vi "Set_To_Idle_State.vi"(6 "Standalone?":bool, 8 "Error In":errorcluster, 9 "GEA2 Reference In":refnum<k24>, 10 "GEA Inputs":T1 {"Destination" format="%.0x"; "Source" format="%.0x"}, 11 "Device Selected":i32) -> (0 "Error Out":errorcluster, 1 "GEA2 Reference Out":refnum<k24>, 3 "Press Power Key":bool)   [LabVIEW 2014]
uses:
  Common/LabVIEW GEA2 Toolkit/LabVIEW_GEA2_Toolkit.lvlibp/type defs/Source_Destination.ctl
  Common/LabVIEW GEA2 Toolkit/LabVIEW_GEA2_Toolkit.lvlibp/type defs/ERD Read Data In.ctl
  Common/LabVIEW GEA2 Toolkit/LabVIEW_GEA2_Toolkit.lvlibp/type defs/Data Type.ctl
  type defs/HEUI Switches.ctl
  Common/LabVIEW GEA2 Toolkit/LabVIEW_GEA2_Toolkit.lvlibp
  C:/Automation/DLLs/PC Tools .NET/GeaCommunication.dll
panel:
  out "Status 2000":string
  # "2015 Dryer: Set to Idle State"
  # "Send Status ERD 2000.\nIf not in Idle (0), press Power key.\nIf in Idle, do nothing."
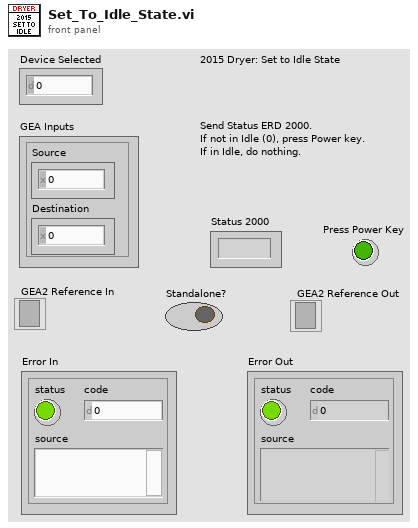
[diagram p1: front panel]
types:
  T1 = typedef "LabVIEW_GEA2_Toolkit.lvlibp/Source_Destination.ctl" = cluster{"Source":u8, "Destination":u8}
  T2 = typedef "LabVIEW_GEA2_Toolkit.lvlibp/ERD Read Data In.ctl" = cluster{"ERD Number":u16, "Data Type":T3}
  T3 = typedef "LabVIEW_GEA2_Toolkit.lvlibp/Data Type.ctl" = enum16{"string", "boolean", "uint8_t", "uint16_t", "uint32_t", "uint64_t", "int8_t", "int16_t", "int32_t", "int64_t"}
  T4 = typedef "LabVIEW_GEA2_Toolkit.lvlibp/ERD Read Data Out.ctl" = cluster{"ERD Number":u16, "Data":string}
  T5 = typedef "HEUI Switches.ctl" = enum16{"Switch Off /  Reset", "SW201 - My Cycle", "SW202 - Delay Dry", "SW203 - Signal / Volume", "SW204 - Damp Alert", "SW205 - Temp", "SW206 - Ext Tumble", "SW207 - Dryness Level", "SW208 -  (-) Time", "SW209 - Time", "SW210 - (+) Time", "SW211 - eDry ", "SW212 - null", "SW213 - Power", "SW214 - Start / Pause"}
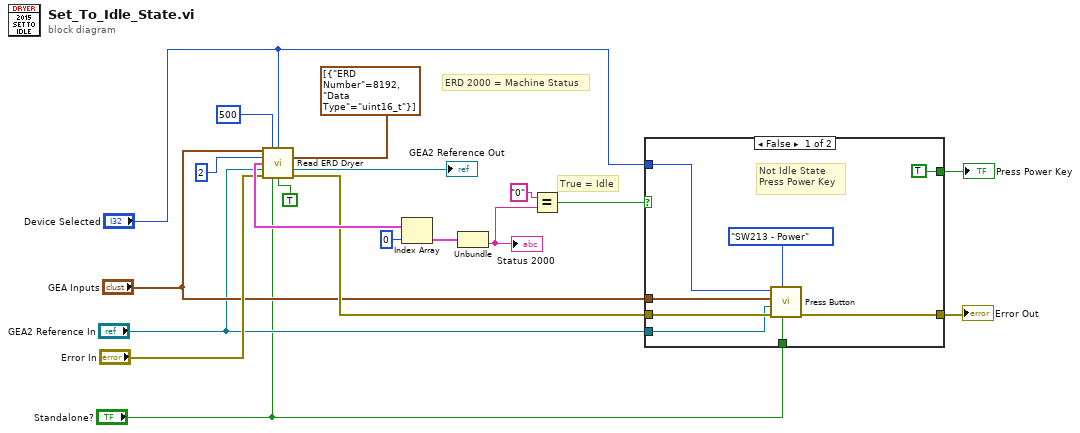
[diagram p0: block diagram]
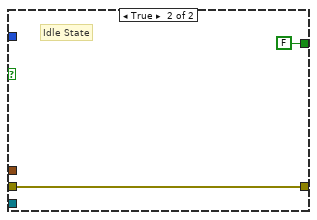
[diagram p2: hidden frame]
diagram:
  # "ERD 2000 = Machine Status"
  # "True = Idle"
  n1 = call "Read ERD Dryer.vi"("GEA Inputs"="GEA Inputs", "Read Timeout (ms)"=u32 500, "Device Selected"="Device Selected", "Retry Count"=2, "Read ERD List"=T2[] [{"ERD Number"=8192, "Data Type"=enum."uint16_t"}], "GEA2 Reference In"="GEA2 Reference In", "Error In"="Error In", "Standalone?"="Standalone?", "Verify ERD Response?"=TRUE) -> ("ERD Data Out"=w14:T4[], "GEA2 Reference Out"=→"GEA2 Reference Out":refnum<k24>, "Error Out"=w7:errorcluster)  [unwired: 3 in, 1 out]
  n2 = Index Array(array=w14, index=0) -> (element=w16:T4)
  n3 = Unbundle(w16) -> ("Data"=w19:string)  [unwired: 1 out]
  "Status 2000" <- w19
  n4 = Equal?(x="0", y=w19) -> (x = y?=w9:bool)
  n5 = case shown="False" w9 {
    tunnel: w7 -> [w27 w29]
    tunnel: [w26 w29] -> w6
    tunnel: [TRUE ("Press Power Key") FALSE ("Press Power Key")] -> w5
    tunnel: "Device Selected" -> [w24 _]
    tunnel: "GEA Inputs" -> [w23 _]
    tunnel: "GEA2 Reference In" -> [w22 _]
    tunnel: "Standalone?" -> [w21 _]
    frame False {
      # "Not Idle State\nPress Power Key"
      n6 = call "Press Button.vi"("Standalone?"=w21, "Button"=HEUI_Switches."SW213 - Power", "Error In"=w27, "GEA2 Reference In"=w22, "GEA Inputs"=w23, "Device Selected"=w24) -> ("Error Out"=w26:errorcluster)  [unwired: 4 in, 1 out]
    }
    frame True {
      # "Idle State"
    }
  }
  "Error Out" <- w6
  "Press Power Key" <- w5
